vi "Set_Volt_AutoScalling_Gen_Control.vi"(0 "VISA Oscilloscope":refnum<visa-resource-name>, 1 "VISA Generator":refnum<visa-resource-name>, 2 "Channel":i32(ring)=1 items=["Channel 1"=1, "Channel 2"=2, "Channel 3"=3, "Channel 4"=4], 3 "Amplitude":dbl=1.0, 4 "DC Offset":dbl, 5 "error in (no error)":errorcluster) -> (14 "VISA Oscilloscope":refnum<visa-resource-name>, 15 "VISA Generator":refnum<visa-resource-name>, 19 "error out":errorcluster)   [LabVIEW 2009]
uses:
  Sum_Abrilader/L0_Sum_Adder Folder/C/Program Files/National Instruments/LabVIEW 2012/instr.lib/Agilent 81150/Agilent 81150.lvlib
  Sum_Abrilader/L0_Sum_Adder Folder/C/Program Files/National Instruments/LabVIEW 2012/instr.lib/Agilent 8000 Series/Agilent 8000 Series.lvlib
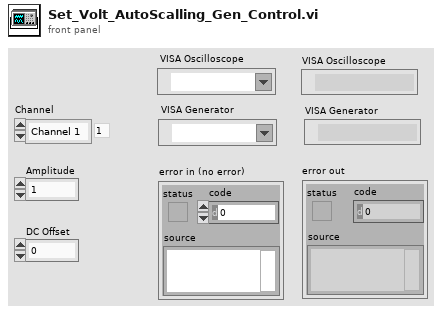
[diagram p1: front panel]
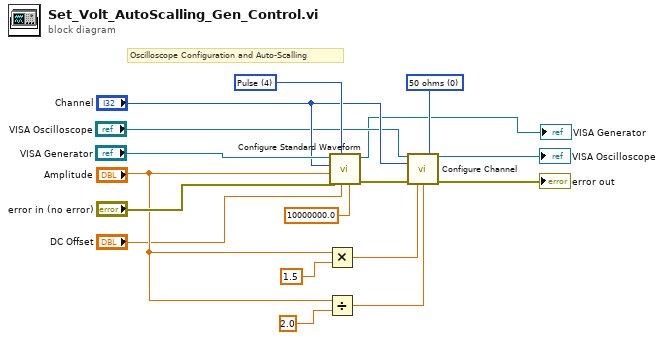
[diagram p0: block diagram]
diagram:
  w10 = u32 0 items=["50 ohms", "1 Mohms"] ("Input Impedance (1: 1 Mohms)")
  w16 = u16 4 items=["Sine", "Square", "Ramp Up", "Ramp Down", "Pulse", "Noise", "DC"] ("Waveform (0: Sine)")
  # "Oscilloscope Configuration and Auto-Scalling"
  n1 = Multiply(x="Amplitude", y=1.5) -> (x*y=w12:dbl)
  n2 = Divide(x="Amplitude", y=2.0) -> (x/y=w11:dbl)
  n3 = call <instrlib>:"Configure Standard Waveform.vi"("Frequency (1000.0 Hz)"=10000000.0, "DC Offset (0.0 Volts)"="DC Offset", "Waveform (0: Sine)"=w16, "error in (no error)"="error in (no error)", "Amplitude (1.0 Vpp)"="Amplitude", "Channel (1: Channel1)"="Channel", "VISA resource name"="VISA Generator") -> ("error out"=w13:errorcluster, "VISA resource name out"=→"VISA Generator":refnum<visa-resource-name>)  [unwired: 3 in]
  n4 = call "Configure Channel.vi"("VISA resource name"="VISA Oscilloscope", "Input Impedance (1: 1 Mohms)"=w10, "Channel (1: Channel 1)"="Channel", "error in (no error)"=w13, "Vertical Range (2.0 V)"=w12, "Vertical Offset (0.0 V)"=w11) -> ("VISA resource name out"=→"VISA Oscilloscope":refnum<visa-resource-name>, "error out"=→"error out":errorcluster)  [unwired: 8 in]
